vi "list cameras.vi"(7 "Enable imaqdx":bool, 8 "error in (no error)":errorcluster) -> (0 "error out":errorcluster, 2 "Cameras":T1[](array[typedef]))   [LabVIEW 2023, in "Vision.lvlib"]
uses:
  Vision.lvlib
  camera.ctl
  camera driver.ctl
  C:/Users/cfangmeier3/Desktop/nebraska-silicon-lab/pixel-gantry-control/Gantry/Shared Components/bin/uEyeDotNet.dll
  bin/uEyeDotNet.dll
  <vilib>/vision/driver/NI_Vision_Acquisition_Software.lvlib
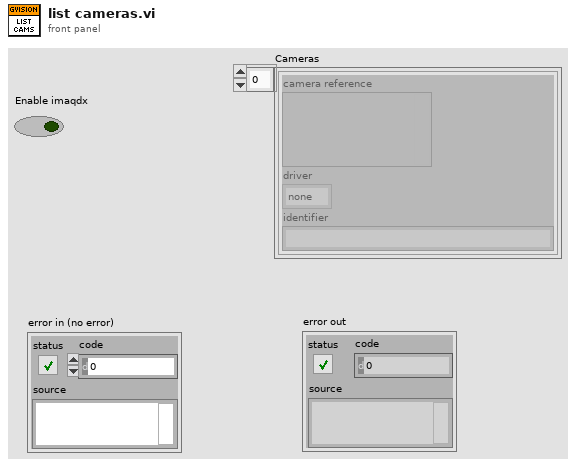
[diagram p1: front panel]
types:
  T1 = typedef "Vision.lvlib/camera.ctl" = cluster{"camera reference":variant, "driver":T2, "identifier":string}
  T2 = typedef "Vision.lvlib/camera driver.ctl" = enum16{"none", "ueye", "wmf", "imaqdx"}
  T3 = cluster{"Type":u32, "Version":u32, "Flags":u32, "SerialNumberHigh":u32, "SerialNumberLow":u32, "BusType":u32, "InterfaceName":string, "VendorName":string, "ModelName":string, "CameraFileName":string, "CameraAttributeURL":string}[]
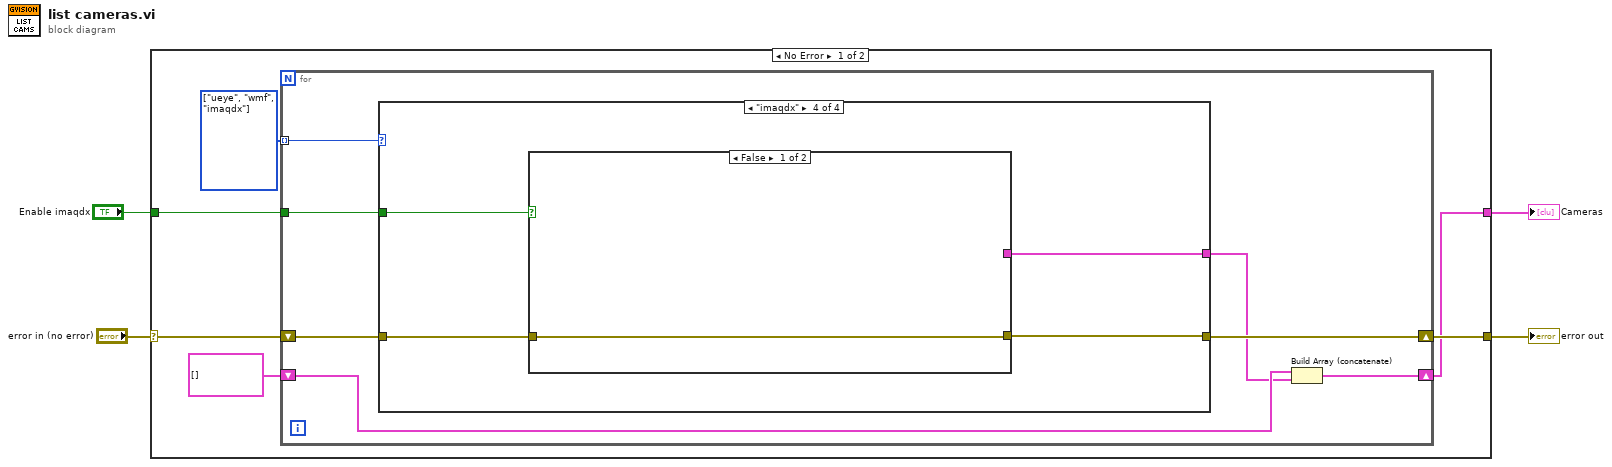
[diagram p0: block diagram]
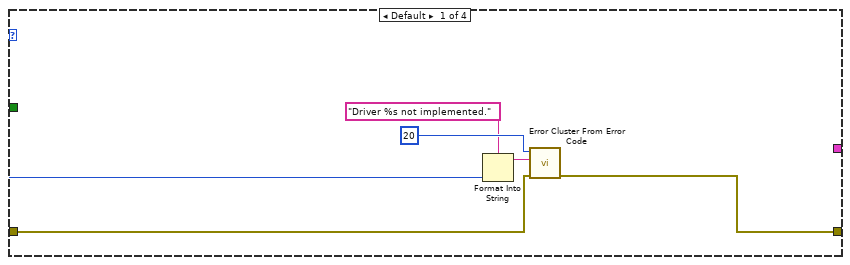
[diagram p2: hidden frame]
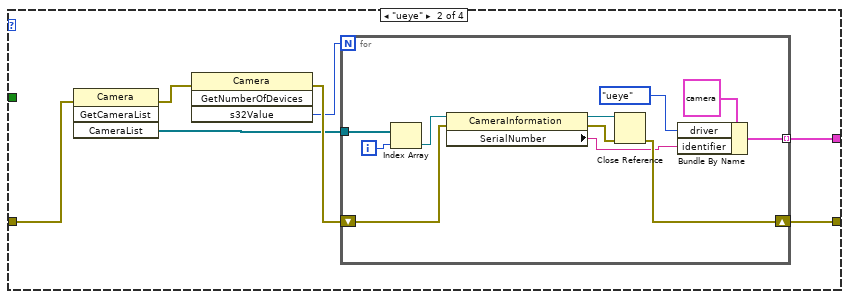
[diagram p3: hidden frame]
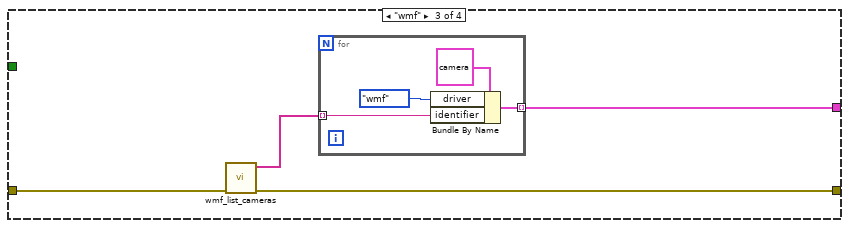
[diagram p4: hidden frame]
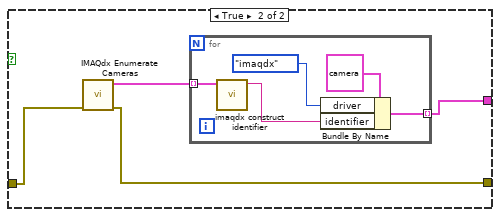
[diagram p5: hidden frame]
diagram:
  n1 = case shown="No Error" "error in (no error)" {
    selector: "error in (no error)" -> [w10 w64]
    tunnel: [w9 w64] -> w3
    tunnel: [w6 _] -> w2
    tunnel: "Enable imaqdx" -> [w5 _]
    frame No Error {
      w8 = T2[] [enum."ueye", enum."wmf", enum."imaqdx"] items=["none", "ueye", "wmf", "imaqdx"]
      n2 = for {
        shift-right: [w16] -> w9
        shift-left: w10 -> [w17]
        tunnel: w8 -> [w15] mode=indexing
        shift-right: [w12] -> w6
        shift-left: T1[] [] -> [w14]
        tunnel: w5 -> [w11]
        n3 = case shown="\"imaqdx\"" w15 {
          selector: w15 -> [w19 _ _ _]
          tunnel: w17 -> [w22 w30 w45 w52]
          tunnel: [w21 w27 w42 w50] -> w16
          tunnel: [_ w24 w43 w51] -> w13
          tunnel: w11 -> [_ _ _ w53]
          frame Default {
            n4 = Format Into String(format string="Driver %s not implemented.", w19) -> (resulting string=w18:string)  [unwired: 2 in, 1 out]
            n5 = call <vilib>:"Error Cluster From Error Code.vi"("error in (no error)"=w22, "error message (\"\")"=w18, "error code (0)"=20) -> ("error out"=w21:errorcluster)  [unwired: 6 in]
          }
          frame "ueye" {
            n6 = invoke on="Methodenknoten" class="Camera" method="GetCameraList"(error in=w30) -> (error out=w29:errorcluster, "CameraList"=w26:refnum<k24>[])  [unwired: 3 in, 2 out]
            n7 = invoke on="Methodenknoten" class="Camera" method="GetNumberOfDevices"(error in=w29) -> (error out=w28:errorcluster, "s32Value"=w25:i32)  [unwired: 3 in, 2 out]
            n8 = for {
              N: w25 -> [_]
              shift-right: [w35] -> w27
              shift-left: w28 -> [w37]
              tunnel: w26 -> [w41]
              tunnel: [w31] -> w24 mode=indexing
              i -> [w40]
              n9 = Index Array(array=w41, index=w40) -> (element=w38:refnum<k24>)
              n10 = property class="CameraInformation"(reference=w38, error in=w37) -> (reference out=w39:refnum<k24>, error out=w36:errorcluster, "SerialNumber"=w34:string)
              n11 = Close Reference(reference=w39, error in (no error)=w36) -> (error out=w35:errorcluster)
              n12 = Bundle By Name(cluster=T1 {"camera reference"=variant, "driver"=enum."none", "identifier"=""}, "driver"=camera_driver."ueye", "identifier"=w34) -> (w31:T1)
            }
          }
          frame "wmf" {
            n13 = call "wmf_list_cameras.vi"("error in (no error)"=w45) -> ("error out"=w42:errorcluster, "Cam Names"=w44:string[])  [unwired: 8 in, 1 out]
            n14 = for {
              tunnel: w44 -> [w47] mode=indexing
              tunnel: [w46] -> w43 mode=indexing
              n15 = Bundle By Name(cluster=T1 {"camera reference"=variant, "driver"=enum."none", "identifier"=""}, "driver"=camera_driver."wmf", "identifier"=w47) -> (w46:T1)
            }
          }
          frame "imaqdx" {
            n16 = case shown="False" w53 {
              tunnel: w52 -> [w54 w58]
              tunnel: [_ w56] -> w51
              tunnel: [w54 w55] -> w50
              frame False {
              }
              frame True {
                n17 = call <vilib>:"IMAQdx Enumerate Cameras.vi"("error in"=w58) -> ("error out"=w55:errorcluster, "Camera Information Array"=w57:T3)  [unwired: 9 in]
                n18 = for {
                  tunnel: w57 -> [w62] mode=indexing
                  tunnel: [w59] -> w56 mode=indexing
                  n19 = call "imaqdx construct identifier.vi"("Camera Information"=w62) -> ("resulting string"=w61:string)  [unwired: 10 in]
                  n20 = Bundle By Name(cluster=T1 {"camera reference"=variant, "driver"=enum."none", "identifier"=""}, "driver"=camera_driver."imaqdx", "identifier"=w61) -> (w59:T1)
                }
              }
            }
          }
        }
        n21 = Build Array (concatenate)(w14, w13) -> (w12:T1[])
      }
    }
    frame Error {
    }
  }
  "error out" <- w3
  "Cameras" <- w2
